vi "RSNRPZ VXIPnp Error Converter.vi"(8 "error in":errorcluster, 10 "VXIPnp error code":i32, 11 "VISA session":refnum<visa-resource-name> caption="VISA resource name") -> (0 "error out":errorcluster, 3 "dup VISA session":refnum<visa-resource-name> caption="VISA resource name")   [LabVIEW 2017]
doc: "This VI converts error codes from VXIPnp instrument driver to standard LabVIEW error codes. If an error is detected the VI builds the appropriate error cluster that is readable by one of the error handlers supplied with LabVIEW."
uses:
  rsnrpz_32.dll
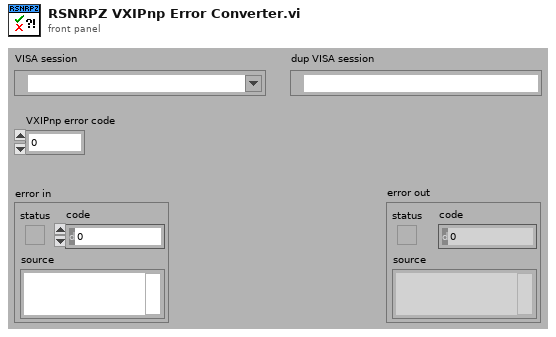
[diagram p1: front panel]
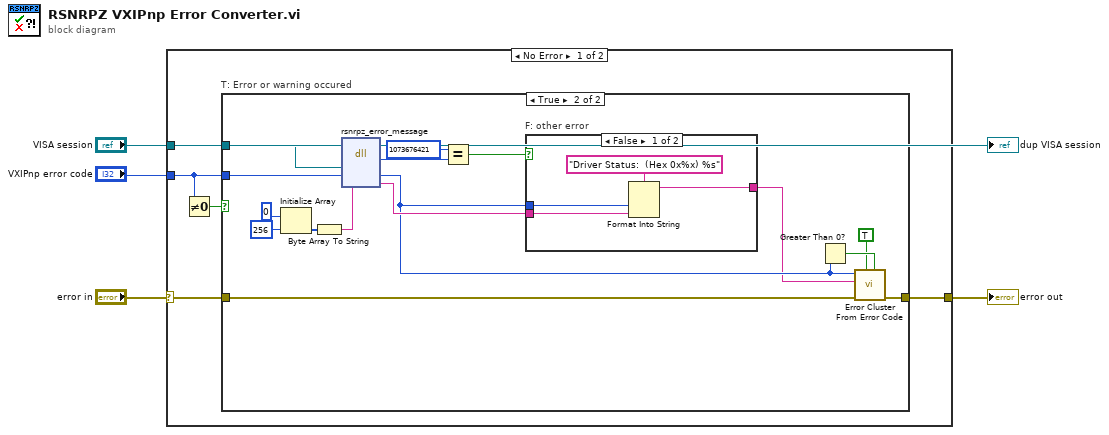
[diagram p0: block diagram]
diagram:
  n1 = case shown="No Error" "error in" {
    selector: "error in" -> [w6 w31]
    tunnel: [w5 w31] -> w1
    tunnel: "VXIPnp error code" -> [w7 _]
    tunnel: "VISA session" -> [w9 _]
    frame No Error {
      n2 = Not Equal To 0?(x=w7) -> (x != 0?=w8:bool)
      n3 = case "T: Error or warning occured" shown="True" w8 {
        tunnel: w7 -> [_ w26]
        tunnel: w9 -> [_ w25]
        tunnel: w6 -> [w10 w16]
        tunnel: [w10 w15] -> w5
        frame False {
        }
        frame True {
          n4 = Initialize Array(u8 0, 256) -> (w23:u8[])
          n5 = Byte Array To String(unsigned byte array=w23) -> (string=w17:string)
          n6 = dll-call lib="C:/Users/labadmin/Documents/Jarvis/user_lib/rsnrpz/rsnrpz_32.dll" fn="rsnrpz_error_message"("instrumentHandle"=w25, "statusCode"=w26, "message"=w17) -> ("return type"=w20:i32, "statusCode"=w12:i32, "message"=w18:string)  [unwired: 4 in, 2 out]
          n7 = Equal?(x=1073676421 ("y"), y=w20) -> (x = y?=w19:bool)
          n8 = case "F: other error" shown="False" w19 {
            tunnel: w18 -> [w29 _]
            tunnel: w12 -> [w30 _]
            tunnel: [w27 _] -> w11
            frame False {
              n9 = Format Into String(format string="Driver Status:  (Hex 0x%x) %s", w30, w29) -> (resulting string=w27:string)  [unwired: 2 in, 1 out]
            }
            frame True {
            }
          }
          n10 = Greater Than 0?(x=w12) -> (x > 0?=w14:bool)
          n11 = call <vilib>:"Error Cluster From Error Code.vi"("is warning? (False)"=w14, "show call chain? (False)"=TRUE, "error in (no error)"=w16, "error message (\"\")"=w11, "error code (0)"=w12) -> ("error out"=w15:errorcluster)  [unwired: 4 in]
        }
      }
    }
    frame Error {
    }
  }
  "error out" <- w1
  "dup VISA session" <- "VISA session"
